vi "Open Tab Refs.vi"() -> ()   [LabVIEW 2020]
panel:
  in  "Tab Control 8":enum32{"Page 1", "Page 2"}(tab)
  in  "Tab Control 7":enum32{"Page 1", "Page 2"}(tab)
  in  "Tab Control 6":enum32{"Page 1", "Page 2"}(tab)
  in  "Tab Control 5":enum32{"Page 1", "Page 2"}(tab)
  out "Refs":refnum<vi>[](array[refnum])
  out "Array 2":string[](array[string])
  in  "Tab Control":enum32{"Page 1", "Page 2"}(tab)
  in  "Tab Control 3":enum32{"Page 1", "Page 2"}(tab)
  in  "Tab Control 4":enum32{"Page 1", "Page 2"}(tab)
  in  "Tab Control 2":enum32{"Page 1", "Page 2"}(tab)
  out "error out":errorcluster
  in  "error in":errorcluster
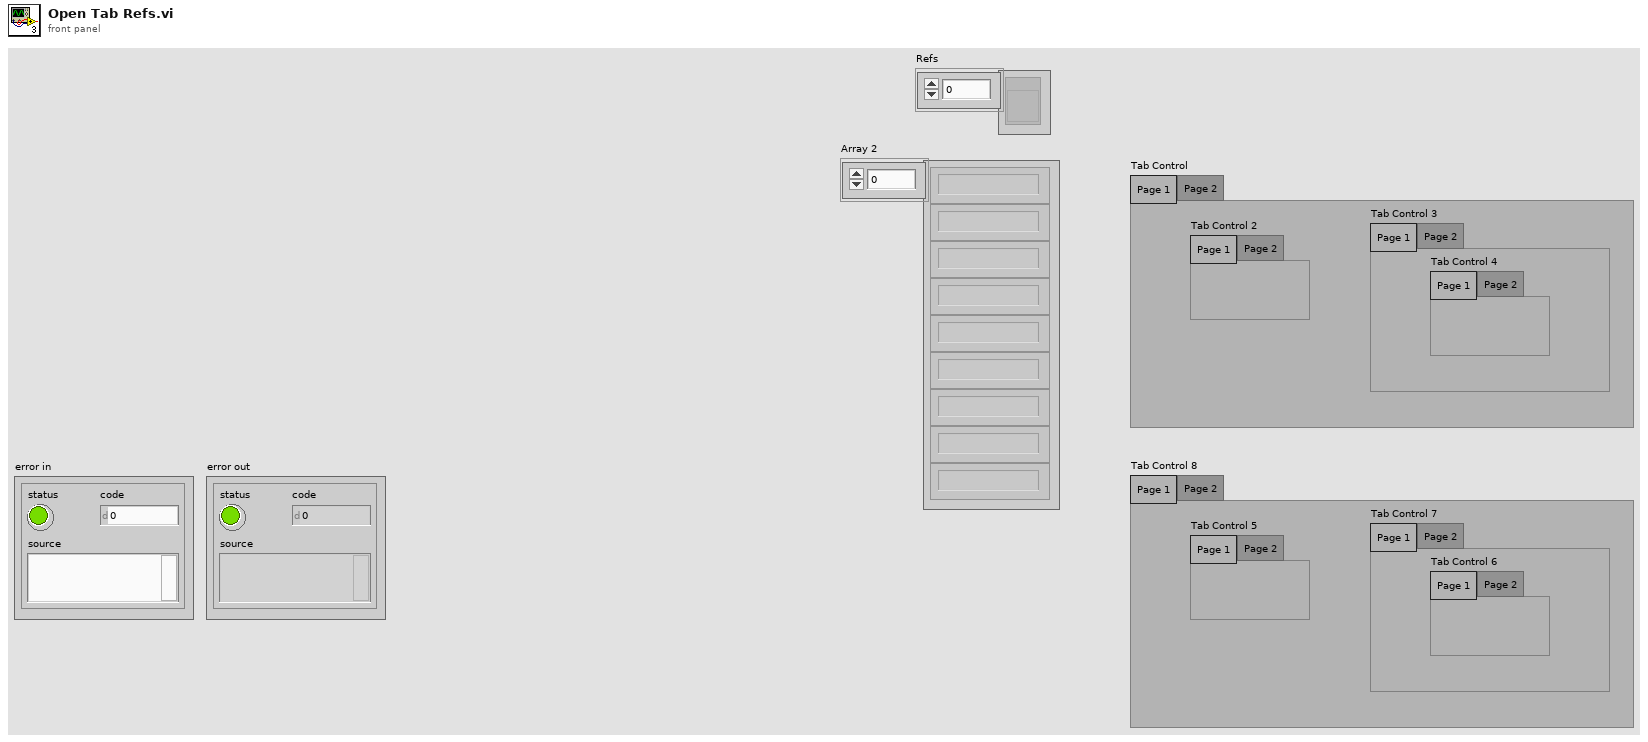
[diagram p1: front panel]
types:
  T1 = typedef "VI Server_RefsCluster.ctl" = cluster{"Labels":string[], "Refs":refnum<vi>[], "VI Ref":refnum<vi>}
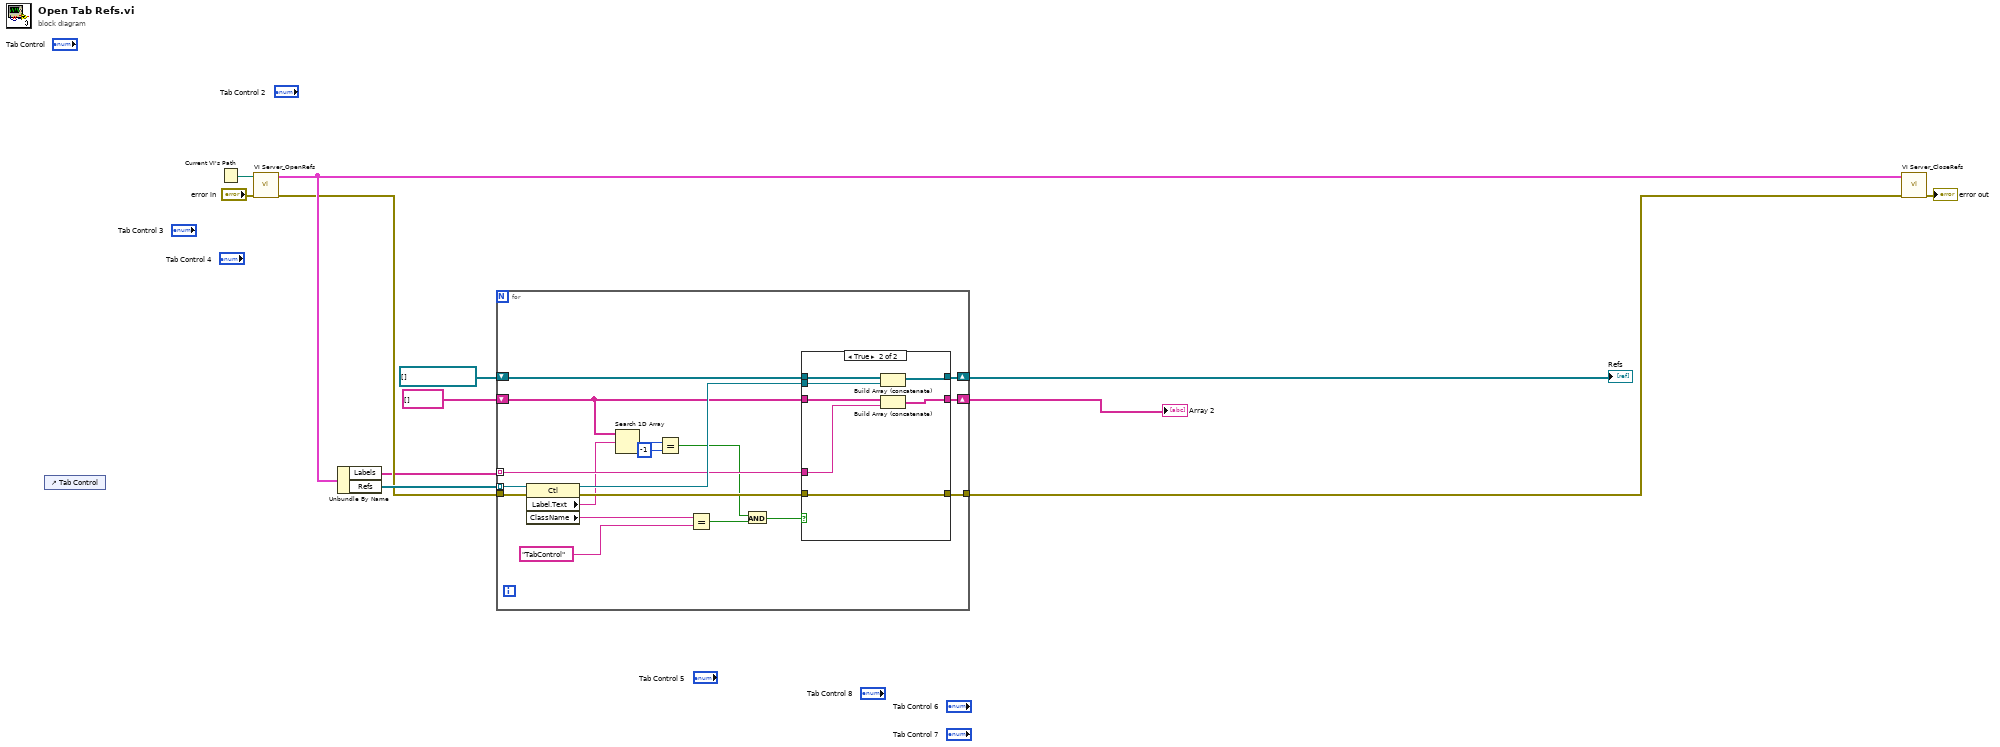
[diagram p0: block diagram]
diagram:
  n1 = control-ref of="Tab Control"() -> ()  [unwired: 1 out]
  n2 = Current VI's Path() -> (path=w12:path)
  n3 = call "VI Server_OpenRefs.vi"("error in"="error in", "VI Path"=w12) -> ("error out"=w7:errorcluster, "VI Server.RefsCluster"=w9:T1)  [unwired: 8 in]
  n4 = Unbundle By Name(w9) -> ("Labels"=w3:string[], "Refs"=w8:refnum<vi>[])
  n5 = for {
    tunnel: w8 -> [w30] mode=indexing
    tunnel: w7 -> [w29]
    tunnel: [w25] -> w6
    shift-right: [w24] -> w4
    shift-left: refnum<vi>[] [] ("Refs") -> [w23]
    tunnel: w3 -> [w21] mode=indexing
    shift-right: [w22] -> w1
    shift-left: string[] [] -> [w19]
    n6 = property class="Ctl"(reference=w30, error in=w29) -> (reference out=w27:refnum<vi>, error out=w26:errorcluster, "Label.Text"=w18:string, "ClassName"=w20:string)
    n7 = Search 1D Array(1D array=w19, element=w18) -> (index of element=w17:i32)  [unwired: 1 in]
    n8 = Equal?(x=w17, y=-1) -> (x = y?=w13:bool)
    n9 = Equal?(x=w20, y="TabControl") -> (x = y?=w15:bool)
    n10 = And(x=w13, y=w15) -> (x .and. y?=w14:bool)
    n11 = case shown="True" w14 {
      tunnel: w27 -> [_ w38]
      tunnel: w26 -> [w32 w40]
      tunnel: [w32 w40] -> w25
      tunnel: w23 -> [w33 w39]
      tunnel: [w33 w37] -> w24
      tunnel: w19 -> [w31 w36]
      tunnel: [w31 w35] -> w22
      tunnel: w21 -> [_ w34]
      frame False {
      }
      frame True {
        n12 = Build Array (concatenate)(w39, w38) -> (w37:refnum<vi>[])
        n13 = Build Array (concatenate)(w36, w34) -> (w35:string[])
      }
    }
  }
  "Array 2" <- w1
  "Refs" <- w4
  n14 = call "VI Server_CloseRefs.vi"("error in"=w6, "VI Server.RefsCluster"=w9) -> ("error out"=→"error out":errorcluster)  [unwired: 9 in]
